vi "PauseMeander.vi"() -> ()   [LabVIEW 2011]
panel:
  out "StopDepthProfile":bool
  out "Pause Meaner":bool
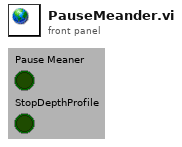
[diagram p1: front panel]
diagram:
